vi "Register Data.vi"(8 "error in (no error)":errorcluster, 11 "UI Controller in":refnum<class "UI Controller.lvclass">) -> (0 "error out":errorcluster, 3 "UI Controller out":refnum<class "UI Controller.lvclass">)   [LabVIEW 2015, in "UI Controller.lvlib" / "UI Controller.lvclass"]
uses:
  UI Controller.lvclass
panel:
  # "NOTICE -- YOU MUST LEAVE THIS NOTICE IN PLACE.\n\nCopyright (c) 2015, LIANG LIU Shawn.Liu.cn@gmail.com\nAll rights reserved.\n\nRedistribution and use in source and binary forms, with or without modification, are permitted provided that the following conditions are met:\n-Redistributions of source code must retain the above copyright notice, this list of conditions and the following disclaimer.\n-Redistributions in binary form must reproduce the above copyright notice, this list of conditions and the following disclaimer in the documentation and/or other materials provided with the distribution.\n-Neither the name of the eLp nor the names of its contributors may be used to endorse or promote products derived from this software without specific prior written permission.\n\nTHIS SOFTWARE IS PROVIDED BY THE COPYRIGHT HOLDERS AND CONTRIBUTORS \"AS IS\" AND ANY EXPRESS OR IMPLIED WARRANTIES, INCLUDING, BUT NOT LIMITED TO, THE IMPLIED WARRANTIES OF MERCHANTABILITY AND FITNESS FOR A PARTICULAR PURPOSE ARE DISCLAIMED. IN NO EVENT SHALL THE COPYRIGHT HOLDER OR CONTRIBUTORS BE LIABLE FOR ANY DIRECT, INDIRECT, INCIDENTAL, SPECIAL, EXEMPLARY, OR CONSEQUENTIAL DAMAGES (INCLUDING, BUT NOT LIMITED TO, PROCUREMENT OF SUBSTITUTE GOODS OR SERVICES; LOSS OF USE, DATA, OR PROFITS; OR BUSINESS INTERRUPTION) HOWEVER CAUSED AND ON ANY THEORY OF LIABILITY, WHETHER IN CONTRACT, STRICT LIABILITY, OR TORT (INCLUDING NEGLIGENCE OR OTHERWISE) ARISING IN ANY WAY OUT OF THE USE OF THIS SOFTWARE, EVEN IF ADVISED OF THE POSSIBILITY OF SUCH DAMAGE."
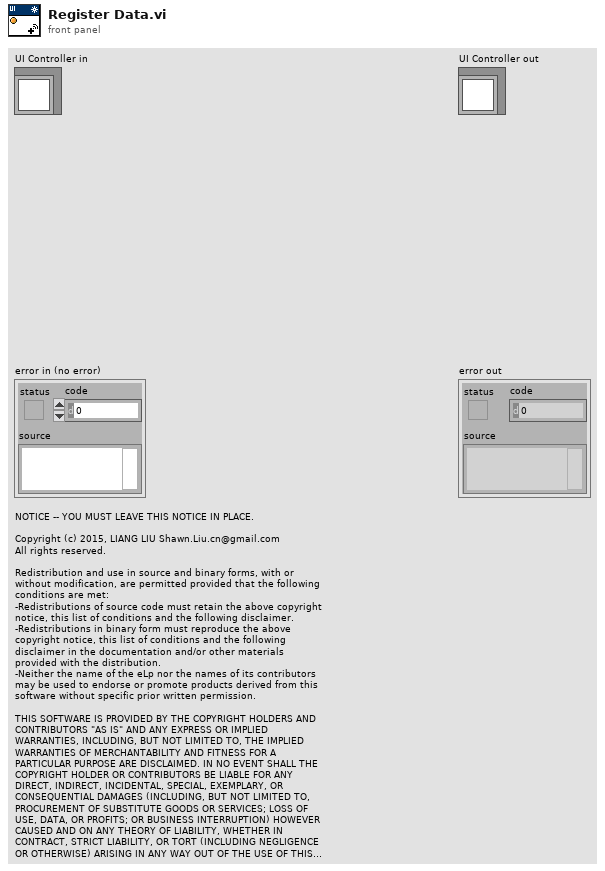
[diagram p1: front panel]
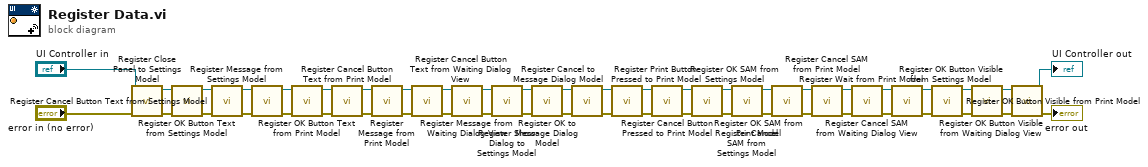
[diagram p0: block diagram]
diagram:
  n1 = call "Register Close Panel to Settings Model.vi"("error in (no error)"="error in (no error)", "UI Controller in"="UI Controller in") -> ("error out"=w46:errorcluster, "UI Controller out"=w47:refnum<class "UI Controller.lvclass">)  [unwired: 8 in]
  n2 = call "Register OK Button Text from Settings Model.vi"("error in (no error)"=w46, "UI Controller in"=w47) -> ("error out"=w44:errorcluster, "UI Controller out"=w45:refnum<class "UI Controller.lvclass">)  [unwired: 8 in]
  n3 = call "Register Cancel Button Text from Settings Model.vi"("error in (no error)"=w44, "UI Controller in"=w45) -> ("error out"=w42:errorcluster, "UI Controller out"=w43:refnum<class "UI Controller.lvclass">)  [unwired: 8 in]
  n4 = call "Register Message from Settings Model.vi"("error in (no error)"=w42, "UI Controller in"=w43) -> ("error out"=w23:errorcluster, "UI Controller out"=w24:refnum<class "UI Controller.lvclass">)  [unwired: 8 in]
  n5 = call "Register OK Button Text from Print Model.vi"("error in (no error)"=w23, "UI Controller in"=w24) -> ("error out"=w27:errorcluster, "UI Controller out"=w28:refnum<class "UI Controller.lvclass">)  [unwired: 8 in]
  n6 = call "Register Cancel Button Text from Print Model.vi"("error in (no error)"=w27, "UI Controller in"=w28) -> ("error out"=w25:errorcluster, "UI Controller out"=w26:refnum<class "UI Controller.lvclass">)  [unwired: 8 in]
  n7 = call "Register Message from Print Model.vi"("error in (no error)"=w25, "UI Controller in"=w26) -> ("error out"=w10:errorcluster, "UI Controller out"=w11:refnum<class "UI Controller.lvclass">)  [unwired: 8 in]
  n8 = call "Register Cancel Button Text from Waiting Dialog View.vi"("error in (no error)"=w10, "UI Controller in"=w11) -> ("error out"=w8:errorcluster, "UI Controller out"=w9:refnum<class "UI Controller.lvclass">)  [unwired: 8 in]
  n9 = call "Register Message from Waiting Dialog View.vi"("error in (no error)"=w8, "UI Controller in"=w9) -> ("error out"=w6:errorcluster, "UI Controller out"=w7:refnum<class "UI Controller.lvclass">)  [unwired: 8 in]
  n10 = call "Register Show Dialog to Settings Model.vi"("error in (no error)"=w6, "UI Controller in"=w7) -> ("error out"=w39:errorcluster, "UI Controller out"=w40:refnum<class "UI Controller.lvclass">)  [unwired: 8 in]
  n11 = call "Register OK to Message Dialog Model.vi"("error in (no error)"=w39, "UI Controller in"=w40) -> ("error out"=w37:errorcluster, "UI Controller out"=w38:refnum<class "UI Controller.lvclass">)  [unwired: 8 in]
  n12 = call "Register Cancel to Message Dialog Model.vi"("error in (no error)"=w37, "UI Controller in"=w38) -> ("error out"=w33:errorcluster, "UI Controller out"=w34:refnum<class "UI Controller.lvclass">)  [unwired: 8 in]
  n13 = call "Register Print Button Pressed to Print Model.vi"("error in (no error)"=w33, "UI Controller in"=w34) -> ("error out"=w31:errorcluster, "UI Controller out"=w32:refnum<class "UI Controller.lvclass">)  [unwired: 8 in]
  n14 = call "Register Cancel Button Pressed to Print Model.vi"("error in (no error)"=w31, "UI Controller in"=w32) -> ("error out"=w29:errorcluster, "UI Controller out"=w30:refnum<class "UI Controller.lvclass">)  [unwired: 8 in]
  n15 = call "Register OK SAM from Settings Model.vi"("error in (no error)"=w29, "UI Controller in"=w30) -> ("error out"=w35:errorcluster, "UI Controller out"=w36:refnum<class "UI Controller.lvclass">)  [unwired: 8 in]
  n16 = call "Register Cancel SAM from Settings Model.vi"("error in (no error)"=w35, "UI Controller in"=w36) -> ("error out"=w21:errorcluster, "UI Controller out"=w22:refnum<class "UI Controller.lvclass">)  [unwired: 8 in]
  n17 = call "Register OK SAM from Print Model.vi"("error in (no error)"=w21, "UI Controller in"=w22) -> ("error out"=w19:errorcluster, "UI Controller out"=w20:refnum<class "UI Controller.lvclass">)  [unwired: 8 in]
  n18 = call "Register Cancel SAM from Print Model.vi"("error in (no error)"=w19, "UI Controller in"=w20) -> ("error out"=w4:errorcluster, "UI Controller out"=w5:refnum<class "UI Controller.lvclass">)  [unwired: 8 in]
  n19 = call "Register Cancel SAM from Waiting Dialog View.vi"("error in (no error)"=w4, "UI Controller in"=w5) -> ("error out"=w2:errorcluster, "UI Controller out"=w3:refnum<class "UI Controller.lvclass">)  [unwired: 8 in]
  n20 = call "Register Wait from Print Model.vi"("error in (no error)"=w2, "UI Controller in"=w3) -> ("error out"=w17:errorcluster, "UI Controller out"=w18:refnum<class "UI Controller.lvclass">)  [unwired: 8 in]
  n21 = call "Register OK Button Visible from Print Model.vi"("error in (no error)"=w17, "UI Controller in"=w18) -> ("error out"=w15:errorcluster, "UI Controller out"=w16:refnum<class "UI Controller.lvclass">)  [unwired: 8 in]
  n22 = call "Register OK Button Visible from Settings Model.vi"("error in (no error)"=w15, "UI Controller in"=w16) -> ("error out"=w13:errorcluster, "UI Controller out"=w14:refnum<class "UI Controller.lvclass">)  [unwired: 8 in]
  n23 = call "Register OK Button Visible from Waiting Dialog View.vi"("error in (no error)"=w13, "UI Controller in"=w14) -> ("error out"=→"error out":errorcluster, "UI Controller out"=→"UI Controller out":refnum<class "UI Controller.lvclass">)  [unwired: 8 in]
